vi "myRIO_BRig DIO 16-bit Bank.vi"(5 "DIO 15:8 Refnum":refnum<k21>, 7 "DIO 7:0 Refnum":refnum<k21>, 8 "OUT 15:0":u16 format="%016b", 11 "DIR 15:0":u16 format="%016b") -> (3 "IN 15:0":u16 format="%016b")   [LabVIEW 2014]
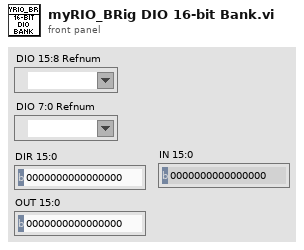
[diagram p1: front panel]
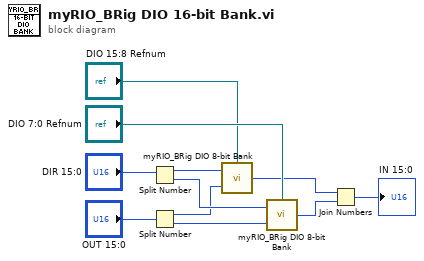
[diagram p0: block diagram]
diagram:
  n1 = Split Number(x="DIR 15:0") -> (hi(x)=w7:u8, lo(x)=w6:u8)
  n2 = Split Number(x="OUT 15:0") -> (hi(x)=w5:u8, lo(x)=w4:u8)
  n3 = call "myRIO_BRig DIO 8-bit Bank.vi"("DIO 7:0 Refnum"="DIO 15:8 Refnum", "OUT 7:0"=w5, "DIR 7:0"=w7) -> ("IN 7:0"=w3:u8)
  n4 = call "myRIO_BRig DIO 8-bit Bank.vi"("DIO 7:0 Refnum"="DIO 7:0 Refnum", "OUT 7:0"=w4, "DIR 7:0"=w6) -> ("IN 7:0"=w2:u8)
  n5 = Join Numbers(hi=w3, lo=w2) -> ((hi.lo)=→"IN 15:0":u16)
